vi "test.vi"() -> ()   [LabVIEW 2010, in "RoiCollection.lvclass"]
uses:
  RoiCollection.lvclass
  common/classes/ImageCollection/ImageCollection/ImageCollection.lvclass
  <vilib>/vision/Image Controls.llb/IMAQ Image.ctl
  common/classes/Image/Image/Image.lvclass
  RoiGeneric/RoiGeneric.lvclass
  RoiEllipsoid/RoiEllipsoid.lvclass
  common/classes/SpaceVector/SpaceVector/SpaceVector.lvclass
panel:
  in  "save ROIs":bool
  in  "quit":bool
  in  "clear ROI":bool
  in  "load ROIs":bool
  in  "load image":bool
  out "z":dbl[unit]
  out "y":dbl[unit]
  out "x":dbl[unit]
  in  "depth":dbl[unit]
  in  "width":dbl[unit]
  in  "length":dbl[unit]
  in  "ROI type":enum16{"ROIGeneric", "ROIEllipsoid"}(ring)
  out "Image":T1(plugin-control)
  in  "depth":dbl[unit](slide)
  # "Test VI for ROICollection"
  # "Calibration"
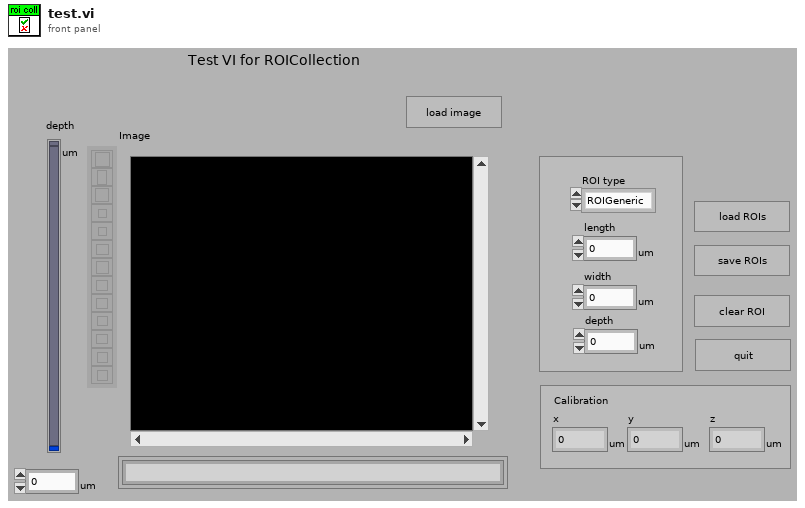
[diagram p1: front panel]
types:
  T1 = typedef "IMAQ Image.ctl" = refnum<image>
  T2 = typedef "Image Type" = u32
  T3 = typedef "eventvkey.ctl" = enum16{"ASCII", "Enter", "Return", "Shift", "Ctrl", "Alt", "Cmd", "Opt", "Caps", "NumLock", "Clear", "Break", "Up", "Down", "Left", "Right", "Insert", "Delete", "Home", "End", "PageUp", "PageDown", "Escape", "Help", "Pause", "ScrollLock", "F1", "F2", "F3", "F4", "F5", "F6", "F7", "F8", "F9", "F10", "F11", "F12", "F13", "F14", "F15", "F16", "F17", "F18", "F19", "F20", "F21", "F22", "F23", "F24", "Play", "VolumeUp", "VolumeDown", "Mute", "Two Byte Char"}
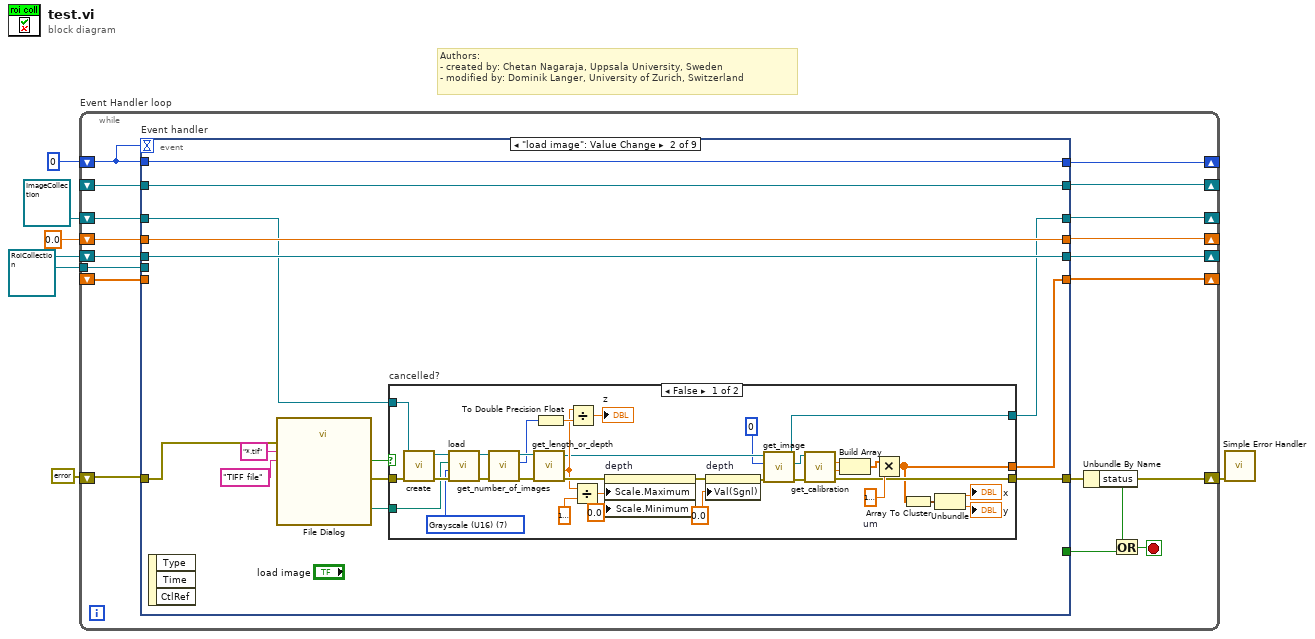
[diagram p0: block diagram]
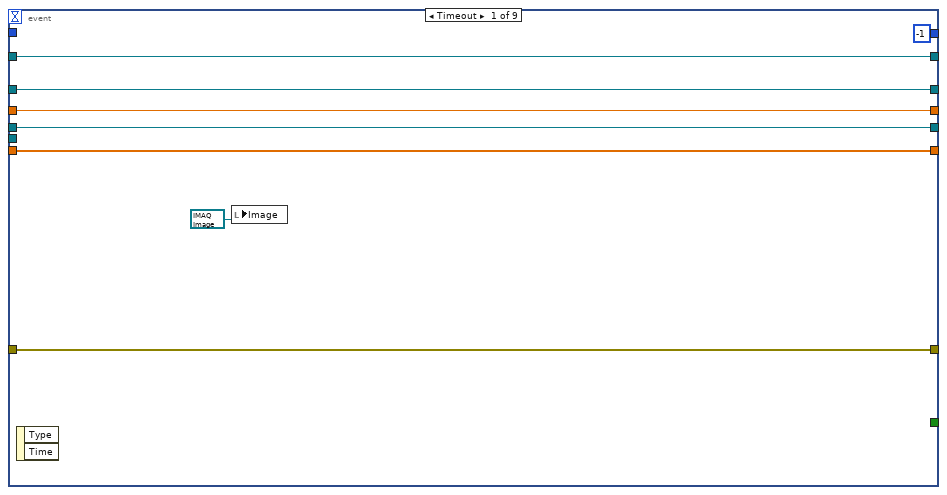
[diagram p2: hidden frame]
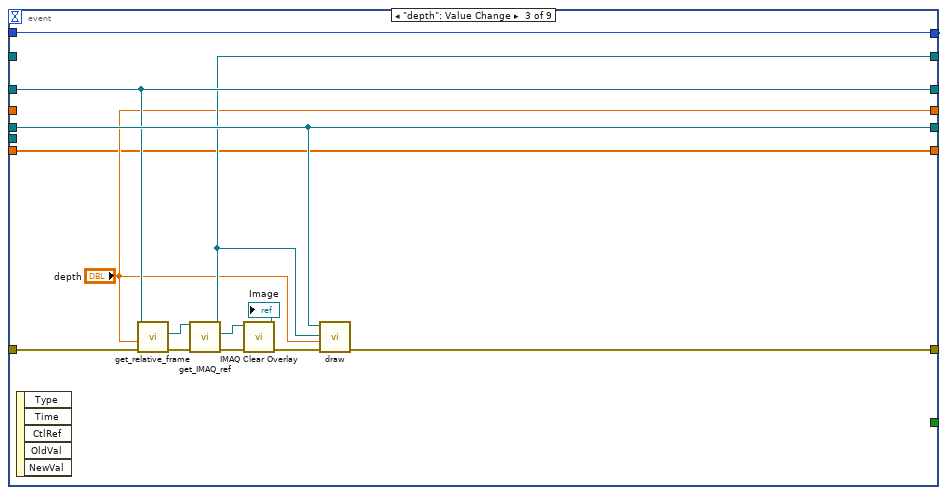
[diagram p4: hidden frame]
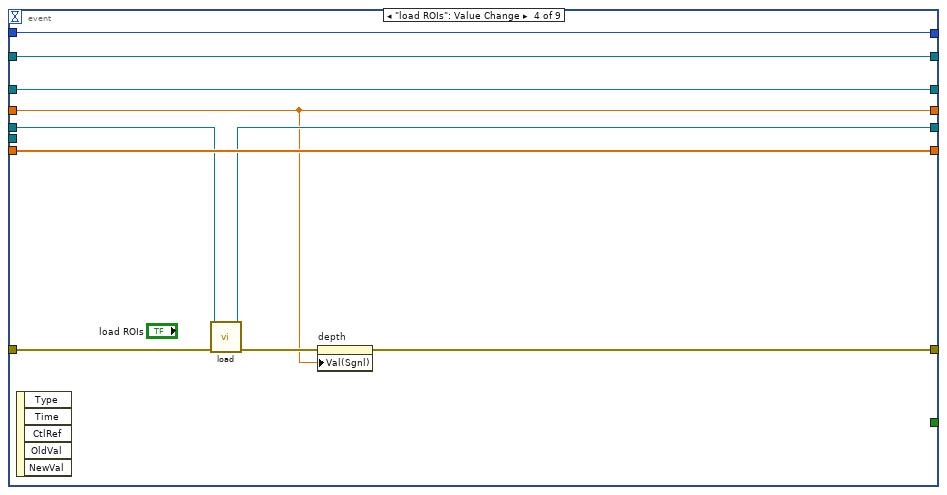
[diagram p5: hidden frame]
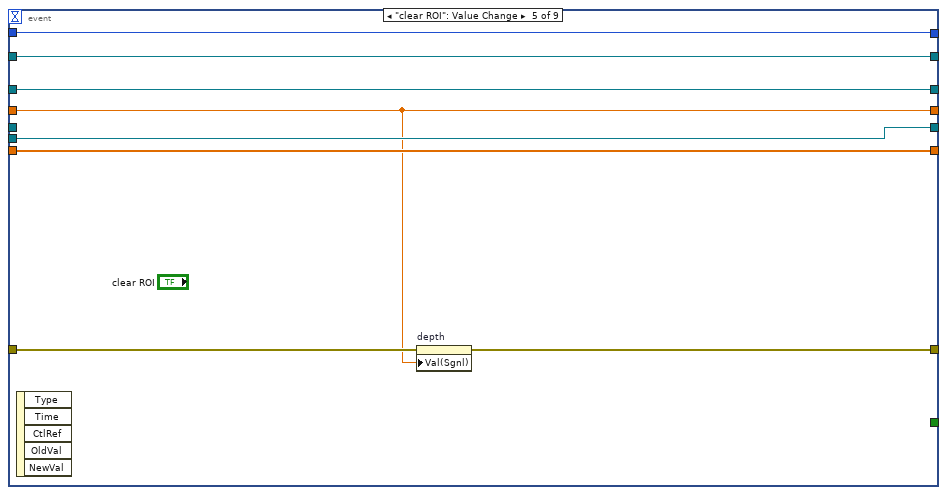
[diagram p6: hidden frame]
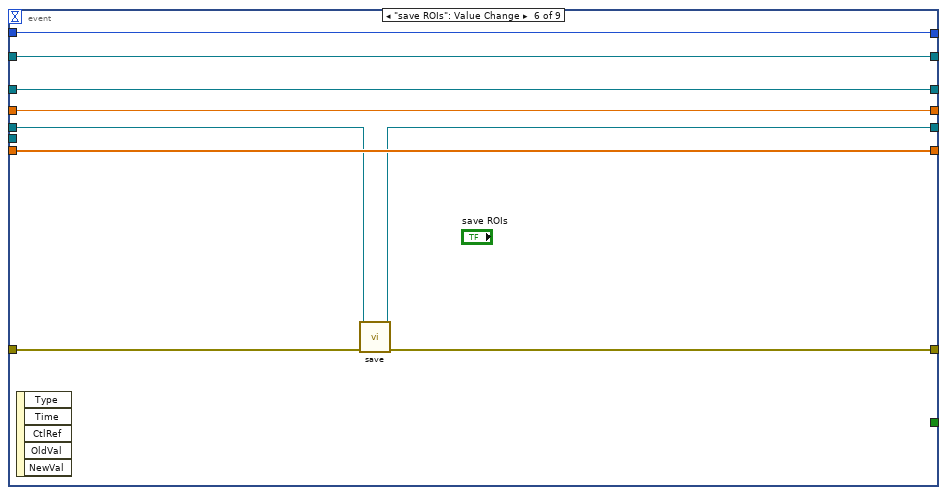
[diagram p7: hidden frame]
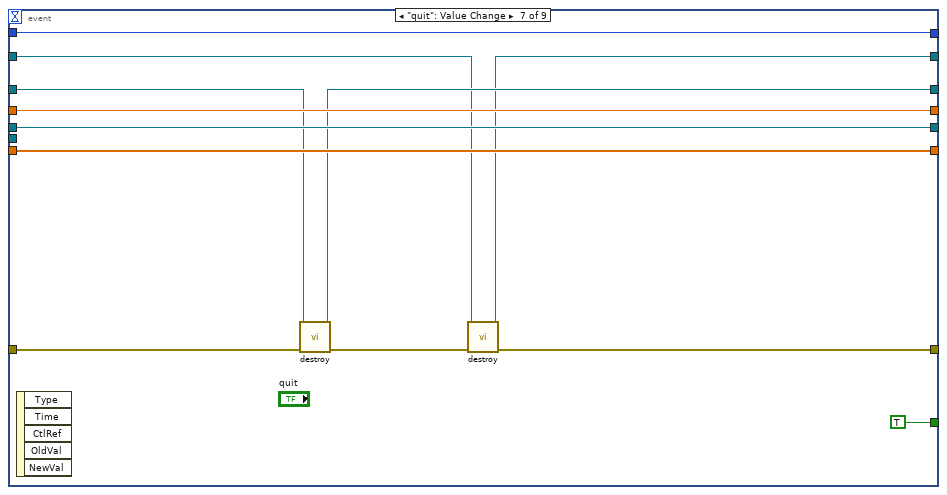
[diagram p8: hidden frame]
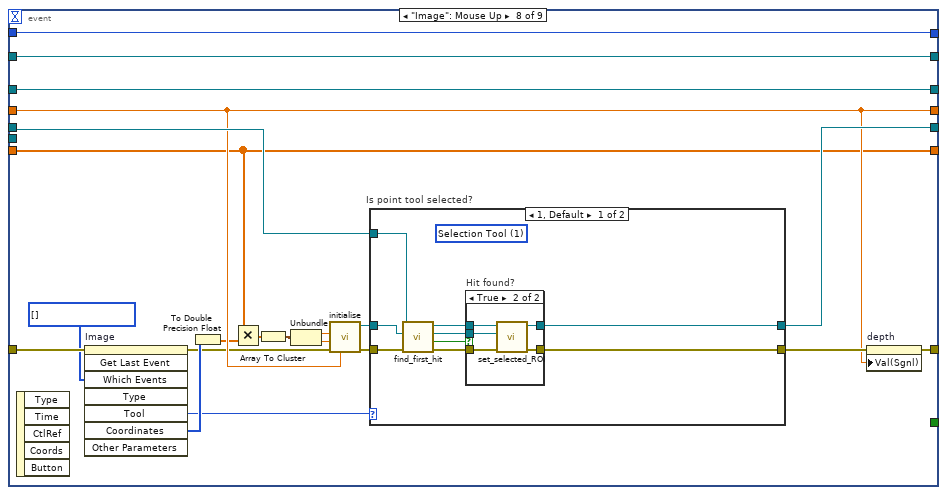
[diagram p9: hidden frame]
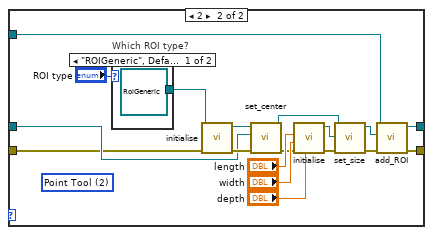
[diagram p11: hidden frame]
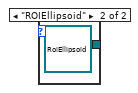
[diagram p12: hidden frame]
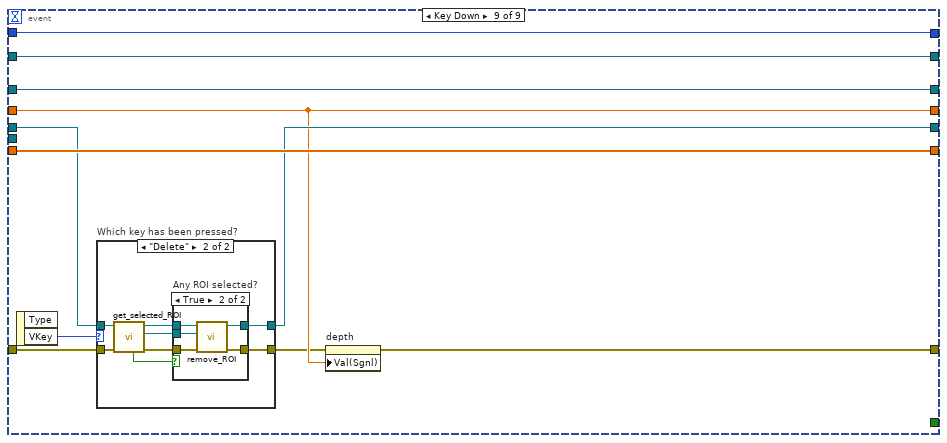
[diagram p13: hidden frame]
diagram:
  w1 = refnum<class "RoiCollection.lvclass"> refnum ("RoiCollection.lvclass")
  # "Authors: \n- created by: Chetan Nagaraja, Uppsala University, Sweden\n- modified by: Dominik Langer, University of Zurich, Switzerland"
  n1 = while "Event Handler loop" {
    shift-right: [w23] -> _
    shift-left: 0 -> [w24]
    shift-right: [w20] -> _
    shift-left: _ -> [w15]
    shift-right: [w19] -> _
    shift-left: refnum<class "ImageCollection.lvclass"> refnum ("ImageCollection.lvclass") -> [w21]
    shift-right: [w18] -> _
    shift-left: dbl[unit] 0.0 ("depth") -> [w16]
    shift-right: [w22] -> _
    shift-left: w1 -> [w7]
    shift-right: [w14] -> _
    shift-left: _ -> [w13]
    shift-right: [w12] -> w2
    shift-left: errorcluster {"status"=FALSE, "code"=0, "source"=""} ("error in") -> [w17]
    tunnel: w1 -> [w8]
    stop <- w9 stop-if-true
    n2 = event "Event handler" shown="[1] \"load image\": Value Change" {
      selector: _ -> [_ _ _ _ _ _ _ _ _]
      dyn-events: _ -> [_ _ _ _ _ _ _ _ _]
      timeout: w24 -> [_ _ _ _ _ _ _ _ _]
      tunnel: w24 -> [_ w46 w95 w107 w115 w124 w136 w157 w204]
      tunnel: [-1 w46 w95 w107 w115 w124 w136 w157 w204] -> w23
      tunnel: w7 -> [w27 w45 w94 w103 _ w118 w135 w149 w198]
      tunnel: [w27 w45 w94 w102 w111 w117 w135 w147 w200] -> w22
      tunnel: w21 -> [w29 w37 w92 w105 w113 w122 w131 w155 w202]
      tunnel: [w30 w44 w89 w106 w114 w123 w128 w156 w203] -> w20
      tunnel: [w29 w36 w92 w105 w113 w122 w130 w155 w202] -> w19
      tunnel: [w28 w43 "depth" w98 w108 w121 w134 w142 w196] -> w18
      tunnel: w17 -> [w31 w42 w91 w101 w110 w116 w127 w154 w199]
      tunnel: [w31 w39 w90 w99 w109 w119 w125 w151 w194] -> w12
      tunnel: w16 -> [w28 w43 _ w98 w108 w121 w134 w142 w196]
      tunnel: w15 -> [w30 w44 _ w106 w114 w123 w129 w156 w203]
      tunnel: [w26 w35 w85 w104 w112 w120 w133 w138 w201] -> w14
      tunnel: w13 -> [w26 _ w85 w104 w112 w120 w133 w138 w201]
      tunnel: [_ _ _ _ _ _ TRUE _ _] -> w10
      tunnel: w8 -> [_ _ _ _ w111 _ _ _ _]
      event Timeout {
        n3 = event-data() -> ()  [unwired: 1 in, 2 out]
        n4 = local write "Image"(T1 refnum ("Image")) -> ()
      }
      event "load image": Value Change {
        n5 = event-data() -> ()  [unwired: 1 in, 3 out]
        n6 = call "File Dialog"("error in"=w42, "pattern (all files)"="*.tif", "pattern label"="TIFF file") -> ("selected path"=w38:path, "cancelled"=w41:bool, "error out"=w40:errorcluster)  [unwired: 9 in, 1 out]
        n7 = case "cancelled?" shown="False" w41 {
          tunnel: w40 -> [w78 w83]
          tunnel: [w51 w83] -> w39
          tunnel: w38 -> [w77 _]
          tunnel: w37 -> [w72 w82]
          tunnel: [w48 w82] -> w36
          tunnel: [w47 _] -> w35
          frame False {
            w58 = dbl[unit] 1e-06  # um
            w76 = T2 7 items=["Grayscale (U8)", "Grayscale (I16)", "Grayscale (SGL)", "Complex (CSG)", "RGB (U32)", "HSL (U32)", "RGB (U64)", "Grayscale (U16)"] ("Image Type")
            n8 = call "create.vi"("error in (no error)"=w78, "ImageCollection in"=w72) -> ("error out"=w79:errorcluster, "ImageCollection out"=w75:refnum<class "ImageCollection.lvclass">)  [unwired: 8 in]
            n9 = call "load.vi"("error in (no error)"=w79, "Image Type"=w76, "path in"=w77, "ImageCollection in"=w75) -> ("error out"=w80:errorcluster, "ImageCollection out"=w74:refnum<class "ImageCollection.lvclass">)  [unwired: 3 in, 3 out]
            n10 = call-dynamic "get_number_of_images.vi"("error in (no error)"=w80, "ImageCollection in"=w74) -> ("error out"=w81:errorcluster, "size"=w71:i32, "ImageCollection out"=w73:refnum<class "ImageCollection.lvclass">)  [unwired: 7 in]
            n11 = call "get_length_or_depth.vi"("error in (no error)"=w81, "ImageCollection in"=w73) -> ("error out"=w68:errorcluster, "total z depth"=w65:dbl[unit], "ImageCollection out"=w50:refnum<class "ImageCollection.lvclass">)  [unwired: 5 in, 2 out]
            n12 = To Double Precision Float(number=w71) -> (double precision float=w70:dbl)
            n13 = Divide(x=w65, y=w70) -> (x/y=→"z":dbl[unit])
            n14 = Divide(x=w65, y=dbl[unit] 1e-06 ("Scale.Range:Minimum")) -> (x/y=w64:dbl)
            n15 = property on="depth" class="Slide (strict)"(error in=w68, "Scale.Maximum"=w64, "Scale.Minimum"=0.0 ("Scale.Range:Minimum")) -> (error out=w63:errorcluster)  [unwired: 1 in, 1 out]
            n16 = property on="depth" class="Slide (strict)"(error in=w63, "Val(Sgnl)"=dbl[unit] 0.0 ("Value (Signaling)")) -> (error out=w52:errorcluster)  [unwired: 1 in, 1 out]
            n17 = call-dynamic "get_image.vi"("error in (no error)"=w52, "index"=0, "ImageCollection in"=w50) -> ("error out"=w55:errorcluster, "Image.lvclass"=w56:refnum<class "Image.lvclass">, "ImageCollection out"=w48:refnum<class "ImageCollection.lvclass">)  [unwired: 6 in]
            n18 = call "get_calibration.vi"("error in (no error)"=w55, "Image.lvclass in"=w56) -> ("error out"=w51:errorcluster, "y"=w60:dbl, "x"=w59:dbl)  [unwired: 4 in, 3 out]
            n19 = Build Array(w59, w60) -> (w57:dbl[])
            n20 = Multiply(x=w57, y=w58) -> (x*y=w47:dbl[unit][])
            n21 = Array To Cluster(array=w47) -> (cluster=w61:cluster{"[0]":dbl[unit], "[1]":dbl[unit]})
            n22 = Unbundle(w61) -> ("[0]"=→"x":dbl[unit], "[1]"=→"y":dbl[unit])
          }
          frame True {
          }
        }
      }
      event "depth": Value Change {
        n23 = event-data() -> ()  [unwired: 1 in, 5 out]
        n24 = call-dynamic "get_relative_frame.vi"("error in (no error)"=w91, "relative depth"="depth", "ImageCollection in"=w92) -> ("error out"=w87:errorcluster, "frame"=w84:refnum<class "Image.lvclass">)  [unwired: 5 in, 2 out]
        n25 = call-dynamic "get_IMAQ_ref.vi"("error in (no error)"=w87, "Image.lvclass in"=w84) -> ("error out"=w97:errorcluster, "Image"=w93:T1, "Image.lvclass out"=w89:refnum<class "Image.lvclass">)  [unwired: 5 in, 2 out]
        n26 = call "IMAQ Clear Overlay"("error in (no error)"=w97, "Image"=w93) -> ("error out"=w86:errorcluster, "Image Out"=→"Image":T1)  [unwired: 8 in]
        n27 = call "draw.vi"("error in (no error)"=w86, "depth"="depth", "Image.lvclass"=w89, "RoiCollection in"=w94) -> ("error out"=w90:errorcluster)  [unwired: 6 in, 1 out]
      }
      event "load ROIs": Value Change {
        n28 = event-data() -> ()  [unwired: 1 in, 5 out]
        n29 = call "load.vi"("error in (no error)"=w101, "RoiCollection in"=w103) -> ("error out"=w100:errorcluster, "RoiCollection out"=w102:refnum<class "RoiCollection.lvclass">)  [unwired: 8 in]
        n30 = property on="depth" class="Slide (strict)"(error in=w100, "Val(Sgnl)"=w98) -> (error out=w99:errorcluster)  [unwired: 1 in, 1 out]
      }
      event "clear ROI": Value Change {
        n31 = event-data() -> ()  [unwired: 1 in, 5 out]
        n32 = property on="depth" class="Slide (strict)"(error in=w110, "Val(Sgnl)"=w108) -> (error out=w109:errorcluster)  [unwired: 1 in, 1 out]
      }
      event "save ROIs": Value Change {
        n33 = event-data() -> ()  [unwired: 1 in, 5 out]
        n34 = call "save.vi"("error in (no error)"=w116, "RoiCollection in"=w118) -> ("error out"=w119:errorcluster, "RoiCollection out"=w117:refnum<class "RoiCollection.lvclass">)  [unwired: 8 in]
      }
      event "quit": Value Change {
        n35 = event-data() -> ()  [unwired: 1 in, 5 out]
        n36 = call-dynamic "destroy.vi"("error in (no error)"=w127, "ImageCollection in"=w131) -> ("error out"=w126:errorcluster, "ImageCollection out"=w130:refnum<class "ImageCollection.lvclass">)  [unwired: 8 in]
        n37 = call-dynamic "destroy.vi"("error in (no error)"=w126, "Image in"=w129) -> ("error out"=w125:errorcluster, "Image out"=w128:refnum<class "Image.lvclass">)  [unwired: 8 in]
      }
      event "Image": Mouse Up {
        w153 = i32[] [] items=["No Event"=0, "Click Event"=1, "Draw Event"=2, "Size Event"=4, "Scroll Event"=5, "Double Click Event"=8]
        n38 = event-data() -> ()  [unwired: 1 in, 5 out]
        n39 = invoke on="Image" class="ImageControl" method="Get Last Event"(error in=w154, "Which Events"=w153) -> (error out=w140:errorcluster, "Tool"=w150:i32, "Coordinates"=w152:i32[])  [unwired: 6 in, 5 out]
        n40 = To Double Precision Float(number=w152) -> (double precision float=w139:dbl[])
        n41 = Multiply(x=w138, y=w139) -> (x*y=w143:dbl[unit][])
        n42 = Array To Cluster(array=w143) -> (cluster=w144:cluster{"[0]":dbl[unit], "[1]":dbl[unit]})
        n43 = Unbundle(w144) -> ("[0]"=w145:dbl[unit], "[1]"=w146:dbl[unit])
        n44 = call "initialise.vi"("z"=w142, "error in (no error)"=w140, "y"=w146, "x"=w145) -> ("error out"=w141:errorcluster, "SpaceVector out"=w137:refnum<class "SpaceVector.lvclass">)  [unwired: 6 in]
        n45 = case "Is point tool selected?" shown="1, Default" w150 {
          tunnel: w141 -> [w165 w175]
          tunnel: [w166 w178] -> w148
          tunnel: w149 -> [w160 w176]
          tunnel: [w161 w174] -> w147
          tunnel: w137 -> [w158 w177]
          frame 1, Default {
            (unwired) 1 items=["None", "Selection Tool", "Point Tool", "Line Tool", "Rectangle Tool", "Oval Tool", "Polygon Tool", "ClosedFreehandTool", "Annulus Tool", "Rotated Rectangle Tool", "Zoom Tool", "Pan Tool", "Polyline Tool", "Freehand Tool"] ("Tool")
            n46 = call "find_first_hit.vi"("error in (no error)"=w165, "SpaceVector.lvclass"=w158, "RoiCollection in"=w160) -> ("error out"=w164:errorcluster, "found?"=w162:bool, "first hit"=w163:refnum<class "RoiGeneric.lvclass">, "RoiCollection out"=w159:refnum<class "RoiCollection.lvclass">)  [unwired: 5 in]
            n47 = case "Hit found?" shown="True" w162 {
              tunnel: [w168 w173] -> w166
              tunnel: w159 -> [w167 w172]
              tunnel: w164 -> [w168 w171]
              tunnel: w163 -> [_ w170]
              tunnel: [w167 w169] -> w161
              frame False {
              }
              frame True {
                n48 = call-dynamic "set_selected_ROI.vi"("error in (no error)"=w171, "RoiGeneric.lvclass"=w170, "RoiCollection in"=w172) -> ("error out"=w173:errorcluster, "RoiCollection out"=w169:refnum<class "RoiCollection.lvclass">)  [unwired: 7 in]
              }
            }
          }
          frame 2 {
            (unwired) 2 items=["None", "Selection Tool", "Point Tool", "Line Tool", "Rectangle Tool", "Oval Tool", "Polygon Tool", "ClosedFreehandTool", "Annulus Tool", "Rotated Rectangle Tool", "Zoom Tool", "Pan Tool", "Polyline Tool", "Freehand Tool"] ("Tool")
            n49 = case "Which ROI type?" shown="\"ROIGeneric\", Default" "ROI type" {
              tunnel: [refnum<class "RoiGeneric.lvclass"> refnum ("RoiGeneric.lvclass") refnum<class "RoiEllipsoid.lvclass"> refnum ("RoiEllipsoid.lvclass")] -> w190
              frame "ROIGeneric", Default {
              }
              frame "ROIEllipsoid" {
              }
            }
            n50 = call-dynamic "initialise.vi"("error in (no error)"=w175, "RoiGeneric in"=w190) -> ("error out"=w188:errorcluster, "RoiGeneric out"=w189:refnum<class "RoiGeneric.lvclass">)  [unwired: 8 in]
            n51 = call-dynamic "set_center.vi"("error in (no error)"=w188, "center"=w177, "RoiGeneric in"=w189) -> ("error out"=w180:errorcluster, "RoiGeneric out"=w182:refnum<class "RoiGeneric.lvclass">)  [unwired: 7 in]
            n52 = call "initialise.vi"("z"="depth", "error in (no error)"=w180, "y"="width", "x"="length") -> ("error out"=w179:errorcluster, "SpaceVector out"=w181:refnum<class "SpaceVector.lvclass">)  [unwired: 6 in]
            n53 = call-dynamic "set_size.vi"("error in (no error)"=w179, "size"=w181, "RoiGeneric in"=w182) -> ("error out"=w186:errorcluster, "RoiGeneric out"=w187:refnum<class "RoiGeneric.lvclass">)  [unwired: 7 in]
            n54 = call "add_ROI.vi"("error in (no error)"=w186, "roi"=w187, "RoiCollection in"=w176) -> ("error out"=w178:errorcluster, "RoiCollection out"=w174:refnum<class "RoiCollection.lvclass">)  [unwired: 7 in]
          }
        }
        n55 = property on="depth" class="Slide (strict)"(error in=w148, "Val(Sgnl)"=w142) -> (error out=w151:errorcluster)  [unwired: 1 in, 1 out]
      }
      event Key Down {
        n56 = event-data() -> ("VKey"=w197:T3)  [unwired: 1 in, 1 out]
        n57 = case "Which key has been pressed?" shown="\"Delete\"" w197 {
          tunnel: [w205 w214] -> w195
          tunnel: [w206 w213] -> w200
          tunnel: w199 -> [w205 w211]
          tunnel: w198 -> [w206 w209]
          frame Default {
          }
          frame "Delete" {
            n58 = call-dynamic "get_selected_ROI.vi"("error in (no error)"=w211, "RoiCollection in"=w209) -> ("error out"=w210:errorcluster, "RoiGeneric.lvclass"=w212:refnum<class "RoiGeneric.lvclass">, "RoiCollection out"=w208:refnum<class "RoiCollection.lvclass">, "any ROI selected?"=w207:bool)  [unwired: 5 in, 1 out]
            n59 = case "Any ROI selected?" shown="True" w207 {
              tunnel: [w216 w221] -> w214
              tunnel: [w215 w220] -> w213
              tunnel: w212 -> [_ w219]
              tunnel: w210 -> [w216 w218]
              tunnel: w208 -> [w215 w217]
              frame False {
              }
              frame True {
                n60 = call "remove_ROI.vi"("error in (no error)"=w218, "RoiGeneric.lvclass"=w219, "RoiCollection in"=w217) -> ("error out"=w221:errorcluster, "RoiCollection out"=w220:refnum<class "RoiCollection.lvclass">)  [unwired: 7 in]
              }
            }
          }
        }
        n61 = property on="depth" class="Slide (strict)"(error in=w195, "Val(Sgnl)"=w196) -> (error out=w194:errorcluster)  [unwired: 1 in, 1 out]
      }
    }
    n62 = Unbundle By Name(w12) -> ("status"=w11:bool)
    n63 = Or(x=w11, y=w10) -> (x .or. y?=w9:bool)
  }
  n64 = call <vilib>:"Simple Error Handler.vi"("error in (no error)"=w2) -> ()  [unwired: 4 in, 5 out]
